vi "ADAM_to_Eng_units.vi"(3 "Ch Description":T1={"Ch Name"="", "Type"="", "Function"=enum."Analogue Input", "Ch State"=enum."On", "Calibration type"=enum."Raw", "A"=0.0, "B"=0.0, "C"=0.0, "D"=0.0, "Comments"="", "Address"={"Main"=0, "Ch."=0, "Sub"=0, "Port Name"=""}, "String"="", "Duty"=65535} {"Duty" format="%.0b"; "D" format="%#_5g"; "C" format="%#_5g"; "B" format="%#_5g"; "A" format="%#_5g"}, 5 "Raw":dbl format="%.2f") -> (1 "Calibrated units":dbl format="%.2f", 2 "Comments":string)   [LabVIEW 2013]
uses:
  ADAM Client/Sub VIs/ADAM Controls/Ch_description_ADAM.ctl
  ADAM Client/Sub VIs/ADAM Controls/Module_type_ADAM.ctl
  ADAM Client/Sub VIs/ADAM Controls/Function_ADAM.ctl
  ADAM Client/Sub VIs/ADAM Controls/Channel_State.ctl
  ADAM Client/Sub VIs/ADAM Controls/Calib_type_ADAM.ctl
  ADAM Client/Sub VIs/ADAM Controls/Address.ctl
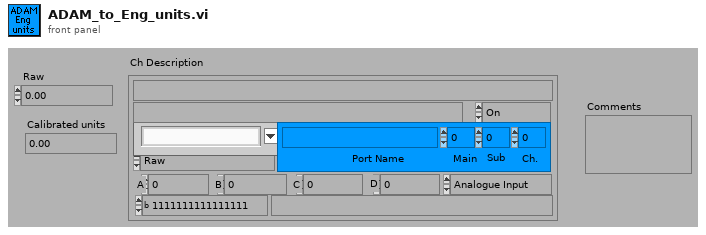
[diagram p1: front panel]
types:
  T1 = typedef "Ch_description_ADAM.ctl" = cluster{"Ch Name":string, "Type":T2, "Function":T3, "Ch State":T4, "Calibration type":T5, "A":dbl, "B":dbl, "C":dbl, "D":dbl, "Comments":string, "Address":T6, "String":string, "Duty":u16}
  T2 = typedef "Module_type_ADAM.ctl" = string
  T3 = typedef "Function_ADAM.ctl" = enum16{"Analogue Input", "Digital Input", "Event counter", "Event rate", "Analogue Output", "Digital Output", "Relay Output"}
  T4 = typedef "Channel_State.ctl" = enum16{"On", "Off", "Always On", "Always Off"}
  T5 = typedef "Calib_type_ADAM.ctl" = enum16{"Raw", "Bx + A", "Cx^2 + Bx + A", "Dx^3 + Cx^2 + Bx + A", "In Band", "Hi-Tec Q", "Hi-Tec M_dot", "Text"}
  T6 = typedef "Address.ctl" = cluster{"Main":i32, "Ch.":i32, "Sub":i32, "Port Name":string}
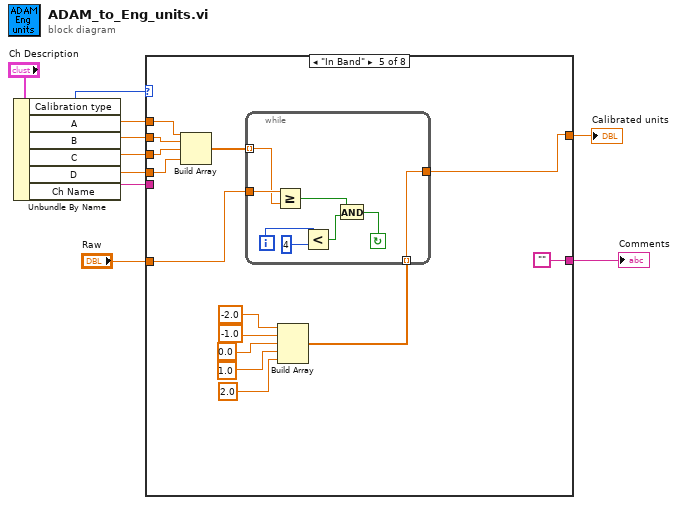
[diagram p0: block diagram]
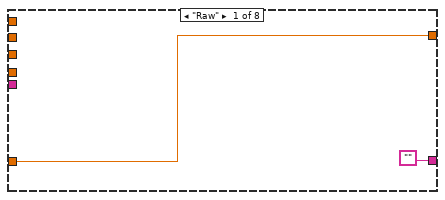
[diagram p2: hidden frame]
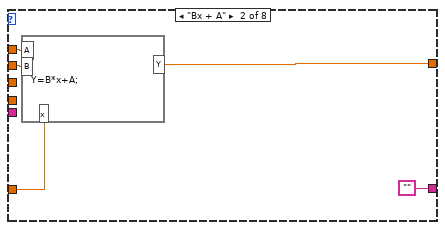
[diagram p3: hidden frame]
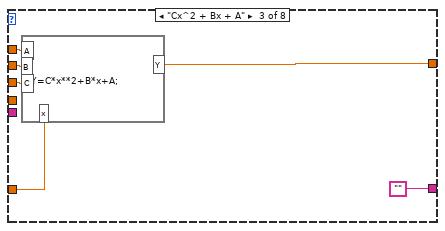
[diagram p4: hidden frame]
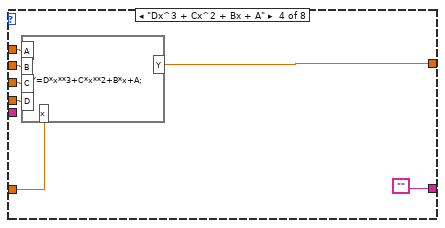
[diagram p5: hidden frame]
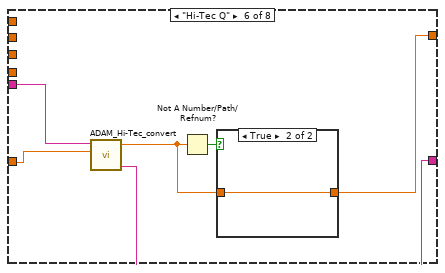
[diagram p6: hidden frame]
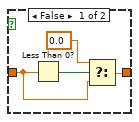
[diagram p7: hidden frame]
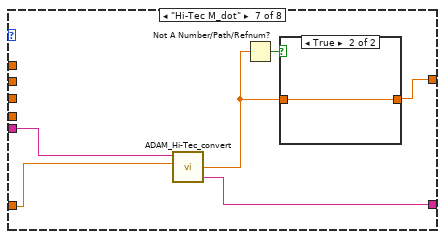
[diagram p8: hidden frame]
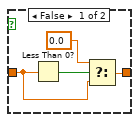
[diagram p9: hidden frame]
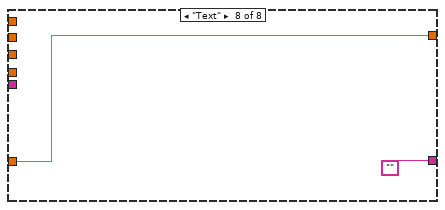
[diagram p10: hidden frame]
diagram:
  n1 = Unbundle By Name("Ch Description") -> ("Calibration type"=w9:T5, "A"=w6:dbl, "B"=w5:dbl, "C"=w4:dbl, "D"=w3:dbl, "Ch Name"=w2:string)
  n2 = case shown="\"In Band\"" w9 {
    tunnel: [w12 w17 w23 w30 w33 w55 w66 w76] -> w8
    tunnel: "Raw" -> [w12 w14 w19 w25 w40 w57 w68 w76]
    tunnel: w6 -> [_ w16 w22 w29 w44 _ _ _]
    tunnel: w5 -> [_ w15 w21 w28 w43 _ _ _]
    tunnel: w4 -> [_ _ w20 w27 w42 _ _ _]
    tunnel: w3 -> [_ _ _ w26 w41 _ _ _]
    tunnel: w2 -> [_ _ _ _ _ w58 w69 _]
    tunnel: ["" "" "" "" "" w53 w64 ""] -> w1
    frame "Raw" {
    }
    frame "Bx + A" {
      n3 = formula code="Y=B*x+A;"("A"=w16, "B"=w15, "x"=w14) -> ("Y"=w17:dbl)
    }
    frame "Cx^2 + Bx + A" {
      n4 = formula code="Y=C*x**2+B*x+A;"("A"=w22, "B"=w21, "C"=w20, "x"=w19) -> ("Y"=w23:dbl)
    }
    frame "Dx^3 + Cx^2 + Bx + A" {
      n5 = formula code="Y=D*x**3+C*x**2+B*x+A;"("A"=w29, "B"=w28, "C"=w27, "D"=w26, "x"=w25) -> ("Y"=w30:dbl)
    }
    frame "In Band" {
      n6 = Build Array(w44, w43, w42, w41) -> (w39:dbl[])
      n7 = Build Array(-2.0, -1.0, 0.0, 1.0, 2.0) -> (w32:dbl[])
      n8 = while {
        tunnel: w32 -> [w50] mode=indexing
        tunnel: [w50] -> w33
        tunnel: w39 -> [w51] mode=indexing
        tunnel: w40 -> [w52]
        i -> [w49]
        stop <- w45 continue-if-true
        n9 = Greater Or Equal?(x=w52, y=w51) -> (x >= y?=w46:bool)
        n10 = Less?(x=w49, y=4) -> (x < y?=w47:bool)
        n11 = And(x=w46, y=w47) -> (x .and. y?=w45:bool)
      }
    }
    frame "Hi-Tec Q" {
      n12 = call "ADAM_Hi-Tec_convert.vi"("Ch Name"=w58, "Raw"=w57) -> ("Q release (l/min)"=w54:dbl, "Comments"=w53:string)  [unwired: 2 in, 2 out]
      n13 = Not A Number/Path/Refnum?(number/path/refnum=w54) -> (NaN/Path/Refnum?=w56:bool)
      n14 = case shown="True" w56 {
        tunnel: [w60 w63] -> w55
        tunnel: w54 -> [w61 w63]
        frame False {
          n15 = Less Than 0?(x=w61) -> (x < 0?=w62:bool)
          n16 = Select(t=0.0, s=w62, f=w61) -> (s? t:f=w60:dbl)
        }
        frame True {
        }
      }
    }
    frame "Hi-Tec M_dot" {
      n17 = call "ADAM_Hi-Tec_convert.vi"("Ch Name"=w69, "Raw"=w68) -> ("M_dot (kg/min)"=w65:dbl, "Comments"=w64:string)  [unwired: 2 in, 2 out]
      n18 = Not A Number/Path/Refnum?(number/path/refnum=w65) -> (NaN/Path/Refnum?=w67:bool)
      n19 = case shown="True" w67 {
        tunnel: [w71 w74] -> w66
        tunnel: w65 -> [w72 w74]
        frame False {
          n20 = Less Than 0?(x=w72) -> (x < 0?=w73:bool)
          n21 = Select(t=0.0, s=w73, f=w72) -> (s? t:f=w71:dbl)
        }
        frame True {
        }
      }
    }
    frame "Text" {
    }
  }
  "Calibrated units" <- w8
  "Comments" <- w1
